vi "icpcon_7005_protocol.vi"(1 "read buffer":string) -> (0 "Data Array":dbl[](array[numeric]))   [LabVIEW 2015]
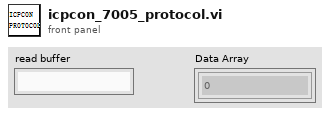
[diagram p1: front panel]
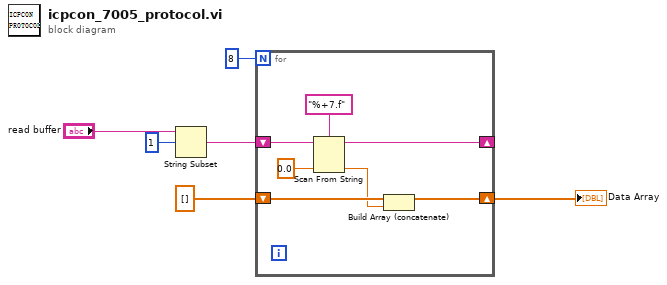
[diagram p0: block diagram]
diagram:
  n1 = String Subset(string="read buffer", offset (0)=1) -> (substring=w3:string)  [unwired: 1 in]
  n2 = for {
    N: 8 -> [_]
    shift-right: [w8] -> _
    shift-left: w3 -> [w12]
    shift-right: [w11] -> w6
    shift-left: dbl[] [] -> [w10]
    n3 = Scan From String(format string="%+7.f", input string=w12, default 1=0.0 ("default value 1")) -> (remaining string=w8:string, output 1=w9:dbl)  [unwired: 2 in, 2 out]
    n4 = Build Array (concatenate)(w10, w9) -> (w11:dbl[])
  }
  "Data Array" <- w6
